vi "ActDriveStraightCalcError-ALT.vi"(10 "Dist (ft)":dbl, 11 "FirstTime":bool) -> (3 "Dist Error (Ft)":dbl)   [LabVIEW 2023]
uses:
  <vilib>/Rock Robotics/Network Tables/NT Write Numeric Array.vi
  <vilib>/Rock Robotics/Network Tables/NT Write Boolean.vi
  <vilib>/Rock Robotics/Network Tables/NT Write Number.vi
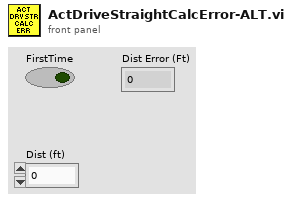
[diagram p1: front panel]
types:
  T1 = typedef "Trajectory_Library.lvlib/SWERVE_DRIVE_MODULE_POSITION.ctl" = cluster{"Distance":dbl, "Angle":T2, "P":bool}
  T2 = typedef "Trajectory_Library.lvlib/ROTATION2D.ctl" = cluster{"VALUE":dbl, "COS":dbl, "SIN":dbl}
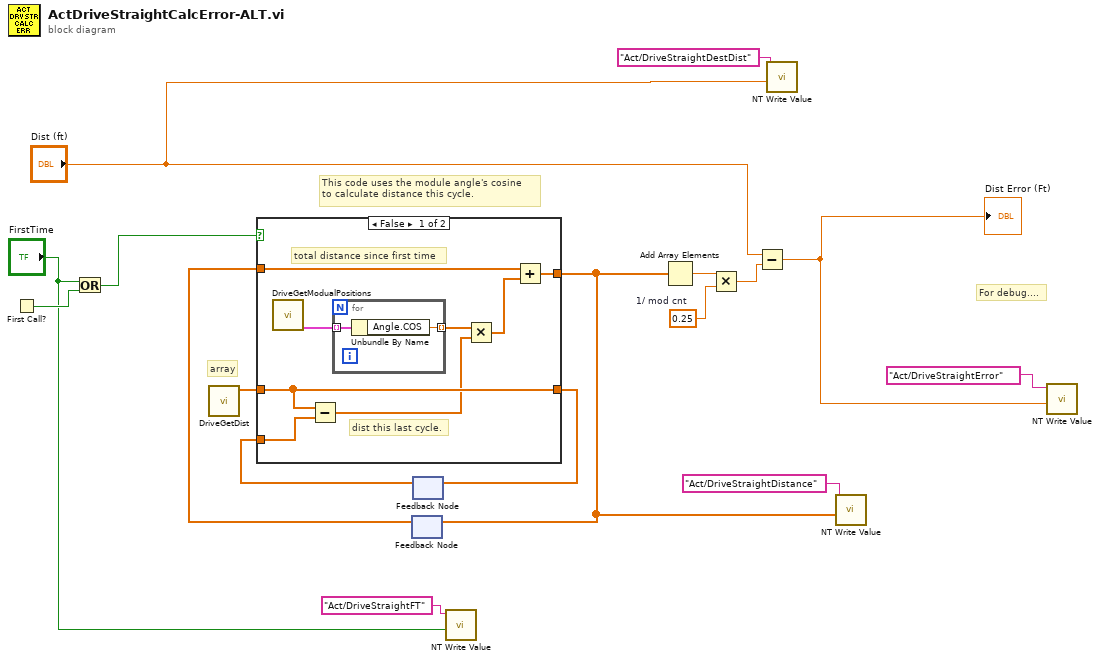
[diagram p0: block diagram]
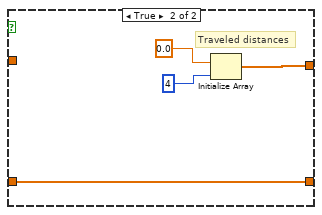
[diagram p2: hidden frame]
diagram:
  w14 = 0.25  # 1/ mod cnt
  # "For debug...."
  # "This code uses the module angle's cosine\nto calculate distance this cycle."
  # "array"
  n1 = First Call?() -> (First Call?: T/F=w10:bool)
  n2 = Or(x="FirstTime", y=w10) -> (x .or. y?=w9:bool)
  n3 = call "DriveGetDist.vi"() -> ("ModuleTravelPosition"=w11:dbl[])  [unwired: 11 in]
  n4 = feedback #1() -> (w15:dbl[])  [unwired: 1 in]
  n5 = feedback #2() -> (w16:dbl[])  [unwired: 1 in]
  n6 = case shown="False" w9 {
    tunnel: w11 -> [w22 w31]
    tunnel: [w22 w31] -> w17
    tunnel: [w24 w28] -> w1
    tunnel: w16 -> [w23 _]
    tunnel: w15 -> [w25 _]
    frame False {
      # "total distance since first time"
      # "dist this last cycle."
      n7 = call "DriveGetModualPositions.vi"() -> ("Swerve_Drive_Modual_Positions"=w18:T1[])  [unwired: 11 in]
      n8 = Subtract(x=w22, y=w23) -> (x-y=w20:dbl[])
      n9 = for {
        tunnel: w18 -> [w27] mode=indexing
        tunnel: [w26] -> w21 mode=indexing
        n10 = Unbundle By Name(w27) -> ("Angle.COS"=w26:dbl)
      }
      n11 = Multiply(x=w21, y=w20) -> (x*y=w19:dbl[])
      n12 = Add(x=w25, y=w19) -> (x+y=w24:dbl[])
    }
    frame True {
      # "Traveled distances"
      n13 = Initialize Array(0.0 ("element"), 4 ("dimension size")) -> (w28:dbl[])
    }
  }
  n14 = feedback-in #1(w1) -> ()
  n15 = feedback-in #2(w17) -> ()
  n16 = call-poly <vilib>:"NT Write Value.vi"("value"="FirstTime", "name"="Act/DriveStraightFT") -> ()  [unwired: 9 in, 1 out]
  n17 = Add Array Elements(numeric array=w1) -> (sum=w13:dbl)
  n18 = Multiply(x=w13, y=w14) -> (x*y=w12:dbl)
  n19 = Subtract(x="Dist (ft)", y=w12) -> (x-y=w3:dbl)
  "Dist Error (Ft)" <- w3
  n20 = call-poly <vilib>:"NT Write Value.vi"("value"="Dist (ft)", "name"="Act/DriveStraightDestDist") -> ()  [unwired: 9 in, 1 out]
  n21 = call-poly <vilib>:"NT Write Value.vi"("value"=w1, "name"="Act/DriveStraightDistance") -> ()  [unwired: 9 in, 1 out]
  n22 = call-poly <vilib>:"NT Write Value.vi"("value"=w3, "name"="Act/DriveStraightError") -> ()  [unwired: 9 in, 1 out]
